vi "Update Tag String.vi"(8 "error in (no error)":errorcluster, 9 "string":string caption="String", 10 "Tag Path":string, 11 "Logger in.lvclass":refnum<class "Logger.lvclass">) -> (0 "error out":errorcluster, 3 "Logger out.lvclass":refnum<class "Logger.lvclass">)   [LabVIEW 2017, in "Logger.lvclass"]
uses:
  Logger.lvclass
  Logger.lvclass/Logger.ctl
  <vilib>/Skyline/Tag/Wrapper/Wrapper_class/Generate Tag Cluster (String) 2.vi
  <vilib>/Skyline/Tag/Wrapper/Wrapper_class/NI Skyline Tag.lvclass
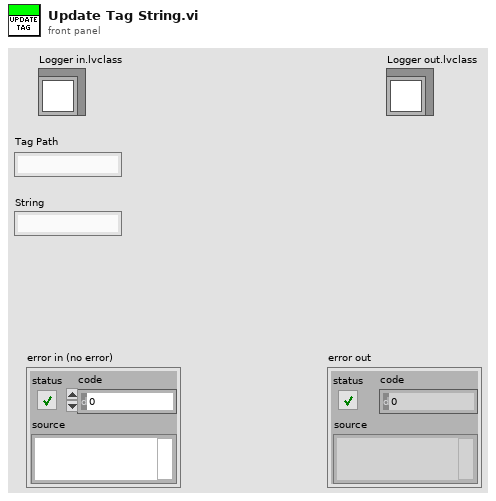
[diagram p1: front panel]
types:
  T1 = cluster{"Tag Units":string, "Tag Path":string, "Waveform":waveform(dbl), "Log":bool, "Tag Reference":refnum<class "NI Skyline Tag.lvclass">}[]
  T2 = typedef "NI Skyline Tag.lvclass/Tag Value Cluster Wrapper.ctl" = cluster{"Configuration":refnum<class "NI Skyline Configuration.lvclass">, "Tag Cluster":T3}
  T3 = typedef "NI Skyline Tag.lvlib/Tag Value Cluster.ctl" = cluster{"Path":string, "Data Type":T4, "Value":string, "Time Stamp":timestamp}
  T4 = typedef "NI Skyline Tag.lvlib/DataType.ctl" = enum32{"Double", "I32", "String", "Boolean", "U64", "Timestamp"}
  T5 = cluster{"Tag Units":string, "Tag Path":string, "Waveform":waveform(dbl), "Log":bool, "Tag Reference":refnum<class "NI Skyline Tag.lvclass">}
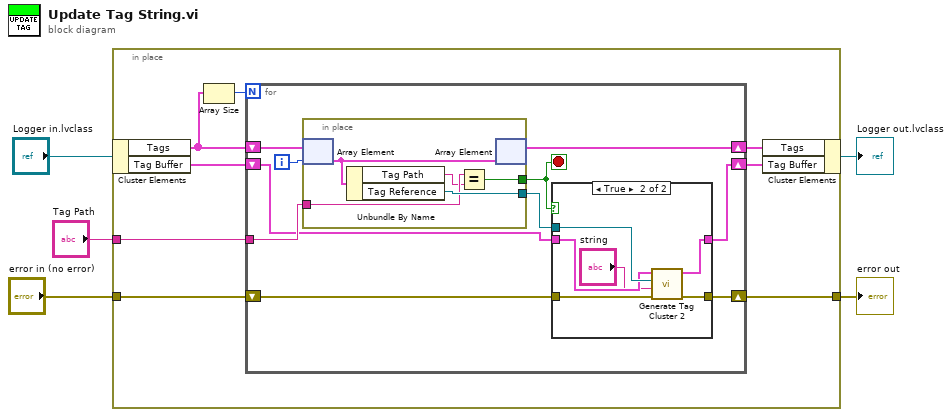
[diagram p0: block diagram]
diagram:
  n1 = in-place {
    in-place-border: "Tag Path" -> [w13]
    in-place-border: "error in (no error)" -> [w7]
    in-place-border: [w6] -> w1
    n2 = in-place-cluster #1("Logger in.lvclass") -> ("Tags"=w10:T1, "Tag Buffer"=w9:T2[])
    n3 = Array Size(array=w10) -> (size(s)=w11:i32)
    n4 = for {
      N: w11 -> [_]
      tunnel: w13 -> [w23]
      shift-right: [w18] -> w12
      shift-left: w10 -> [w22]
      shift-right: [w16] -> w8
      shift-left: w9 -> [w17]
      shift-right: [w14] -> w6
      shift-left: w7 -> [w15]
      i -> [w21]
      stop <- w20 stop-if-true
      n5 = in-place {
        in-place-border: w23 -> [w33]
        in-place-border: [w34] -> w20
        in-place-border: [w36] -> w19
        n6 = in-place-array #2(w22, w21) -> (w35:T5)
        n7 = Unbundle By Name(w35) -> ("Tag Path"=w32:string, "Tag Reference"=w36:refnum<class "NI Skyline Tag.lvclass">)
        n8 = Equal?(x=w33, y=w32) -> (x = y?=w34:bool)
        n9 = in-place-array #2(w35) -> (w18:T1)  [unwired: 1 out]
      }
      n10 = case shown="True" w20 {
        tunnel: w19 -> [_ w31]
        tunnel: w17 -> [w25 w29]
        tunnel: [w25 w30] -> w16
        tunnel: w15 -> [w24 w28]
        tunnel: [w24 w27] -> w14
        frame False {
        }
        frame True {
          n11 = call-poly <vilib>:"Generate Tag Cluster 2.vi"("error in (no error)"=w28, "value"="string", "tag in"=w31, "tag clusters in"=w29) -> ("error out"=w27:errorcluster, "tag clusters out"=w30:T2[])  [unwired: 5 in, 1 out]
        }
      }
    }
    n12 = in-place-cluster #1("Tags"=w12, "Tag Buffer"=w8) -> (→"Logger out.lvclass":refnum<class "Logger.lvclass">)
  }
  "error out" <- w1
